vi "TDMS Write Single Type.vi"(8 "error in (no error)":errorcluster, 9 "Data":dbl[][](array[numeric]), 10 "Timestamps":timestamp[][](array[timestamp]), 11 "Path":path) -> (0 "error out":errorcluster, 2 "Time for Write (S)":dbl, 3 "Path Out":path)   [LabVIEW 2017, in "labview-standard-library.lvlib" / "data-logging.lvlib"]
doc: "Changes the timestamp data to match the data datatype. This eliminates fragmentation as an issue."
uses:
  data-logging.lvlib
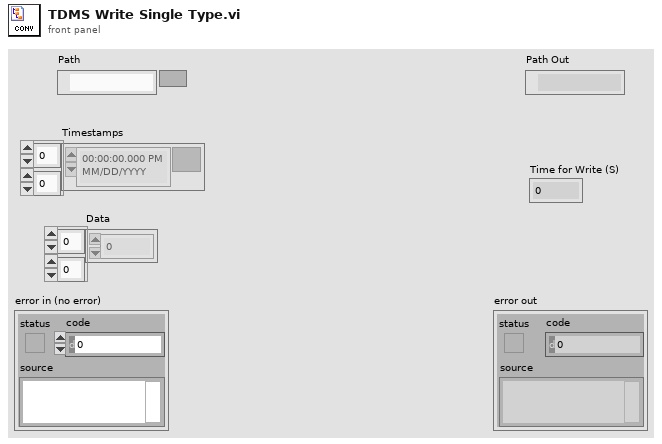
[diagram p1: front panel]
types:
  T1 = enum16{"open", "open or create", "create or replace", "create", "open (read-only)"}
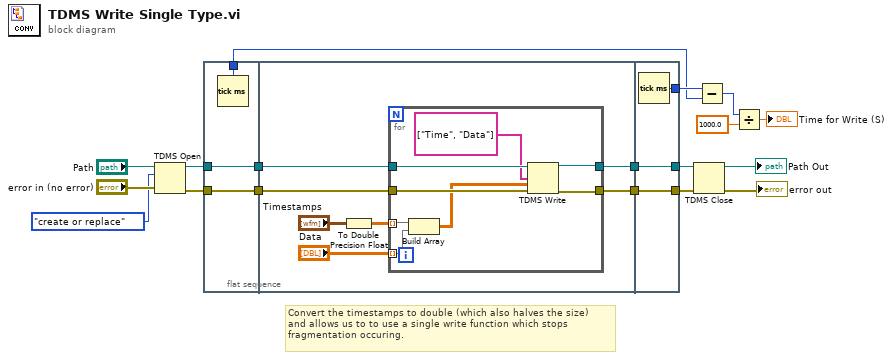
[diagram p0: block diagram]
diagram:
  # "Convert the timestamps to double (which also halves the size)\nand allows us to to use a single write function which stops\nfragmentation occuring."
  n1 = TDMS Open(8:"error in (no error)", 10:T1."create or replace" ("operation (0:open)"), 11:"Path") -> (0:w13:errorcluster, 3:w15:refnum<k34>)  [unwired: 4 in]
  n2 = flat-sequence {
    tunnel: [w21] -> w16
    tunnel: w15 -> [w21]
    tunnel: [w20] -> w14
    tunnel: w13 -> [w20]
    tunnel: [w19] -> w5
    tunnel: w16 -> [w26]
    tunnel: w14 -> [w25]
    tunnel: [w24] -> w8
    tunnel: [w23] -> w7
    tunnel: [w38] -> w11
    tunnel: [w39] -> w12
    tunnel: w8 -> [w39]
    tunnel: w7 -> [w38]
    tunnel: [w37] -> w6
    frame #0 {
      n3 = Tick Count (ms)() -> (millisecond timer value=w19:u32)
    }
    frame #1 {
      n4 = To Double Precision Float(number="Timestamps") -> (double precision float=w22:dbl[][])
      n5 = for {
        tunnel: w22 -> [w31] mode=indexing
        tunnel: "Data" -> [w30] mode=indexing
        tunnel: w26 -> [w36]
        tunnel: w25 -> [w35]
        tunnel: [w33] -> w24
        tunnel: [w32] -> w23
        n6 = Build Array(w31, w30) -> (w29:dbl[][])
        n7 = TDMS Write(0:w36, 7:string[] ["Time", "Data"] ("channel name(s) in (Untitled)"), 9:w29, 11:w35) -> (4:w33:refnum<k34>, 15:w32:errorcluster)  [unwired: 2 in, 2 out]
      }
    }
    frame #2 {
      n8 = Tick Count (ms)() -> (millisecond timer value=w37:u32)
    }
  }
  n9 = TDMS Close(8:w11, 11:w12) -> (0:→"error out":errorcluster, 3:→"Path Out":path)
  n10 = Subtract(x=w6, y=w5) -> (x-y=w4:u32)
  n11 = Divide(x=w4, y=1000.0) -> (x/y=→"Time for Write (S)":dbl)
